vi "Get SMO HELP getAll.vi"(8 "error in (no error)":errorcluster, 11 "Instrument in":refnum<class "Instrument.lvclass">) -> (0 "error out":errorcluster, 1 "response info table":string[][](array[string])=[["name", "description"], ["*", "*"]], 2 "response cluster":variant, 3 "Instrument out":refnum<class "Instrument.lvclass">)   [LabVIEW 2019, in "Instrument.lvclass"]
uses:
  Instrument.lvclass
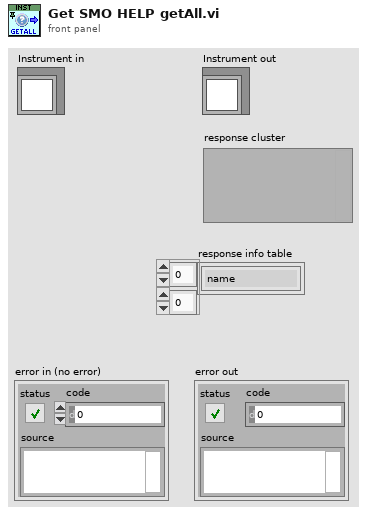
[diagram p1: front panel]
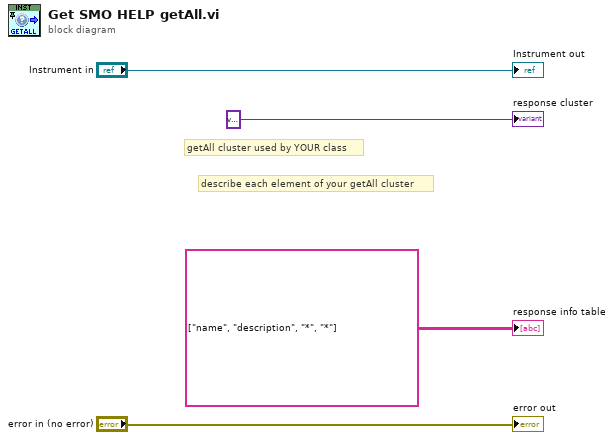
[diagram p0: block diagram]
diagram:
  # "describe each element of your getAll cluster"
  # "getAll cluster used by YOUR class"
  "Instrument out" <- "Instrument in"
  "response info table" <- string[][] [["name", "description"], ["*", "*"]] ("response/request info table: description of request or reponse cluster")
  "error out" <- "error in (no error)"
  "response cluster" <- variant
